vi "MotorOpenCOM.vi"(3 "COM Port in":refnum<visa-resource-name>, 9 "error in (no error)":errorcluster) -> (0 "COM Port out":refnum<visa-resource-name>, 2 "Version":string, 6 "error out":errorcluster)   [LabVIEW 2009]
uses:
  <vilib>/Instr/_visa.llb/VISA Configure Serial Port (Serial Instr).vi
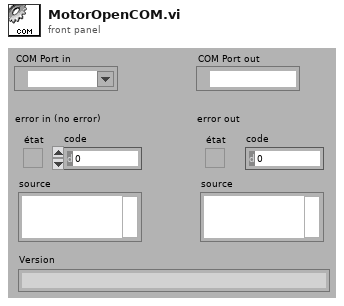
[diagram p1: front panel]
types:
  T1 = enum16{"SEL", "INIT", "MVT", "VMIN", "VMAX", "ACC", "POS", "MPAS", "INT", "JEU", "OFFSET", "L", "B", "STOP"}
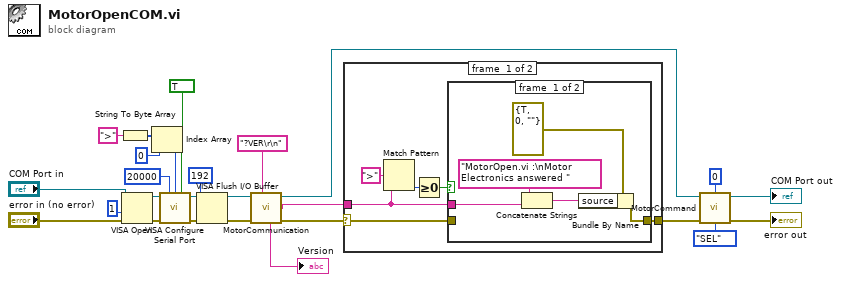
[diagram p0: block diagram]
diagram:
  n1 = String To Byte Array(string=">") -> (unsigned byte array=w18:u8[])
  n2 = VISA Open(access mode=u32 1 ("mode d'accès"), error in (no error)="error in (no error)", VISA resource name="COM Port in") -> (VISA resource name=w14:refnum<visa-resource-name>, error out=w13:errorcluster)  [unwired: 2 out]
  n3 = Index Array ("Indexer un tableau")(array=w18, index=0 ("indice")) -> (element=w16:u8)
  n4 = call-poly "VISA Configure Serial Port"("VISA resource name"=w14, "timeout (10sec)"=u32 20000, "termination char\n(0xA = '\\n' = LF)"=w16, "Enable Termination\nChar (T)"=TRUE ("Enable Termination\nChar (T)"), "error in (no error)"=w13) -> ("VISA resource name out"=w21:refnum<visa-resource-name>, "error out"=w20:errorcluster)  [unwired: 4 in, 5 out]
  n5 = VISA Flush I/O Buffer(VISA resource name=w21, mask (16)=u16 192 ("masque (16)"), error in (no error)=w20) -> (VISA resource name out=w4:refnum<visa-resource-name>, error out=w5:errorcluster)
  n6 = call "MotorCommunication.vi"("Question"="?VER\r\n" ("buffer à écrire"), "error out"=w5, "COM Port in"=w4) -> ("error IO"=w2:errorcluster, "COM Port out"=w3:refnum<visa-resource-name>, "Answer"=w1:string)  [unwired: 4 out]
  "Version" <- w1
  n7 = case shown="No Error" w2 {
    selector: w2 -> [w25 w37]
    tunnel: w1 -> [w27 _]
    tunnel: [w26 w37] -> w12
    frame #0 {
      n8 = Match Pattern(string=w27, regular expression=">" ("expression")) -> (offset past match=w29:i32)  [unwired: 4 out]
      n9 = Greater Or Equal To 0?(x=w29) -> (x >= 0?=w28:bool)
      n10 = case shown="False" w28 {
        tunnel: w25 -> [_ w36]
        tunnel: [w34 w36] -> w26
        tunnel: w27 -> [w35 _]
        frame #0 {
          n11 = Concatenate Strings("MotorOpen.vi :\nMotor Electronics answered " ("source"), w35) -> (w32:string)
          n12 = Bundle By Name(cluster=errorcluster {"status"=TRUE, "code"=0, "source"=""} ("error out"), "source"=w32) -> (w34:errorcluster)
        }
        frame #1 {
        }
      }
    }
    frame #1 {
    }
  }
  "error out" <- w12
  n13 = call "MotorCommand.vi"("Parameter"=0, "COM Port in"=w3, "Command"=T1."SEL", "entrée d'erreur"=w12) -> ("COM Port out"=→"COM Port out":refnum<visa-resource-name>)  [unwired: 5 out]
